vi "Read Interface.lvclass.vi"(8 "error in (no error)":errorcluster, 11 "RxTx in":refnum<class "RxTx.lvclass">) -> (0 "error out":errorcluster, 2 "Interface.lvclass":refnum<class "Interface.lvclass">, 3 "RxTx out":refnum<class "RxTx.lvclass">)   [LabVIEW 2018]
uses:
  RxTx.lvclass
  Interface/Interface.lvclass
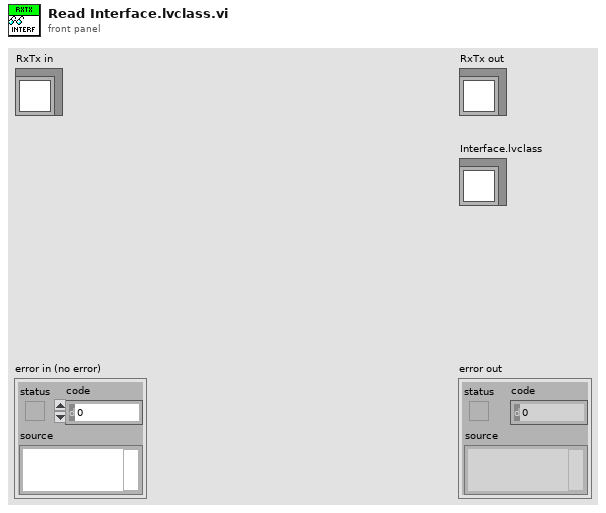
[diagram p1: front panel]
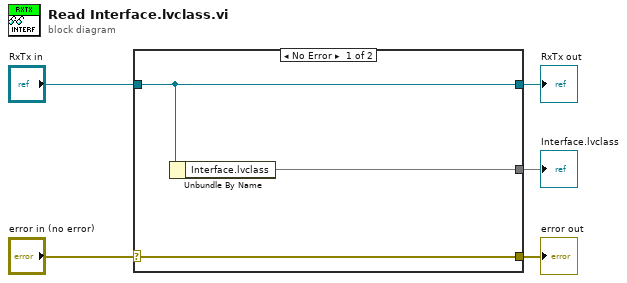
[diagram p0: block diagram]
diagram:
  n1 = case shown="No Error" "error in (no error)" {
    selector: "error in (no error)" -> [w8 w9]
    tunnel: [w8 w9] -> w4
    tunnel: [w7 w10] -> w2
    tunnel: "RxTx in" -> [w7 w10]
    tunnel: [w6 _] -> w1
    frame No Error {
      n2 = Unbundle By Name(w7) -> ("Interface.lvclass"=w6)
    }
    frame Error {
    }
  }
  "error out" <- w4
  "RxTx out" <- w2
  "Interface.lvclass" <- w1
